vi "Close Session.vi"(8 "error in (no error)":errorcluster, 11 "Session in":refnum<class "Plugin Session.lvclass">) -> (0 "error out":errorcluster)   [LabVIEW 2023, in "InstrumentStudio Plugin SDK.lvlib" / "Plugin Session.lvclass"]
doc: "Call this VI to close out all references created for the session and unregister the plugin session with the framework. It should be called at the end of your plugin VI after the event loop is completed as the last call in the VI."
uses:
  Plugin Session.lvclass
  Plugin Session.lvclass/Plugin Session.ctl
  Plugin Events.ctl
  Event Registration Refnum.ctl
  Read Plugin Events.vi
  Read Event Refnum.vi
  InstrumentStudio Plugin SDK.lvlib
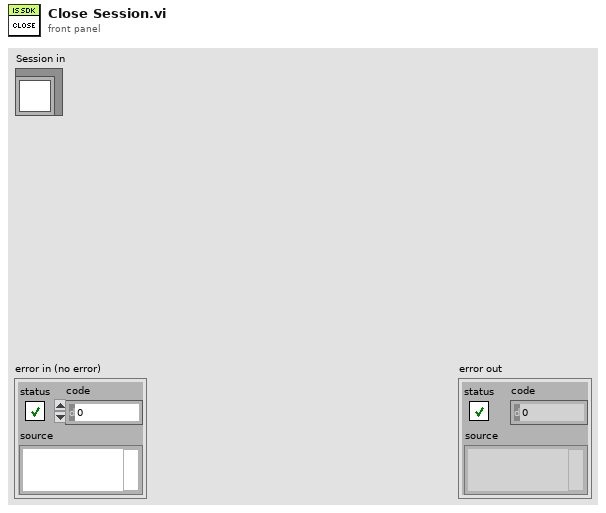
[diagram p1: front panel]
types:
  T1 = typedef "InstrumentStudio Plugin SDK.lvlib/Plugin Events.ctl" = cluster{"Shutdown":refnum<user-event>, "Project Saved":refnum<user-event>, "Stop All Outputs":refnum<user-event>}
  T2 = typedef "InstrumentStudio Plugin SDK.lvlib/Event Registration Refnum.ctl" = refnum<event-registration>
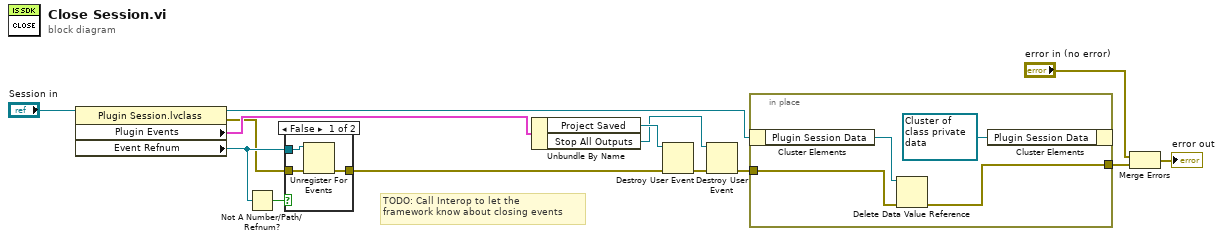
[diagram p0: block diagram]
diagram:
  # "TODO: Call Interop to let the\nframework know about closing events"
  n1 = property class="Plugin Session.lvclass"(reference="Session in") -> (reference out=w2:refnum<class "Plugin Session.lvclass">, error out=w1:errorcluster, "Plugin Events"=w11:T1, "Event Refnum"=w8:T2)  [unwired: 1 in]
  n2 = Not A Number/Path/Refnum?(number/path/refnum=w8) -> (NaN/Path/Refnum?=w12:bool)
  n3 = case shown="False" w12 {
    tunnel: [w17 w18] -> w7
    tunnel: w8 -> [w16 _]
    tunnel: w1 -> [w15 w18]
    frame False {
      n4 = Unregister For Events(event registration refnum=w16, error in=w15) -> (error out=w17:errorcluster)
    }
    frame True {
    }
  }
  n5 = Unbundle By Name(w11) -> ("Project Saved"=w10:refnum<user-event>, "Stop All Outputs"=w9:refnum<user-event>)
  n6 = Destroy User Event(user event=w10, error in=w7) -> (error out=w13:errorcluster)
  n7 = Destroy User Event(user event=w9, error in=w13) -> (error out=w6:errorcluster)
  n8 = in-place {
    in-place-border: w6 -> [w22]
    in-place-border: [w20] -> w3
    n9 = in-place-cluster #1(w2) -> ("Plugin Session Data"=w21:refnum<data-value>)
    n10 = Delete Data Value Reference(data value reference=w21, error in=w22) -> (error out=w20:errorcluster)  [unwired: 1 out]
    n11 = in-place-cluster #1("Plugin Session Data"=refnum<data-value> refnum) -> ()  [unwired: 1 out]
  }
  n12 = Merge Errors("error in (no error)", w3) -> (→"error out":errorcluster)
